vi "DrawSurface.vi"(0 "Surface":T1={"Row Interval"=1.0, "Col Interval"=1.0, "Base"=1.0, "Color Box"=1703680, "Alpha"=1.0}, 1 "Name":string="Surface", 2 "path":path, 3 "error in (no error)":errorcluster) -> (5 "object out":refnum<vi>, 7 "error out":errorcluster)   [LabVIEW 2017]
uses:
  <vilib>/picture/3D Picture Control/Object/Create Object (name).vi
  <vilib>/picture/3D Picture Control/NI_3D Picture Control.lvlib
panel:
  out "Color":T2={"Red"=1.0, "Green"=0.0, "Blue"=0.0, "Alpha"=1.0}
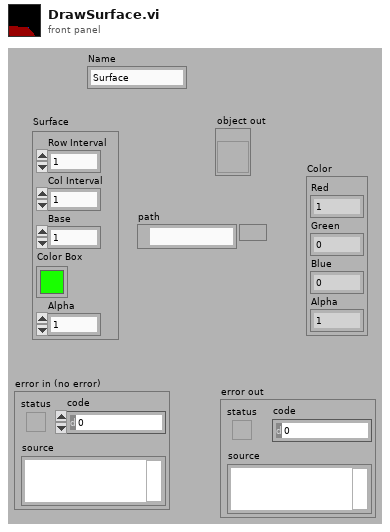
[diagram p1: front panel]
types:
  T1 = cluster{"Row Interval":sgl, "Col Interval":sgl, "Base":sgl, "Color Box":u32, "Alpha":sgl}
  T2 = cluster{"Red":sgl, "Green":sgl, "Blue":sgl, "Alpha":sgl}
  T3 = typedef "QT_Image.ctl" = cluster{"Width":i32, "Height":i32, "Depth":i32, "data":u8[], "Compressed data":u8[], "Color table":u32[], "Duration":i32, "Options":i32, "Timestamp":i32, "ID":i32, "Reserved":i32, "Dialogs":u32}
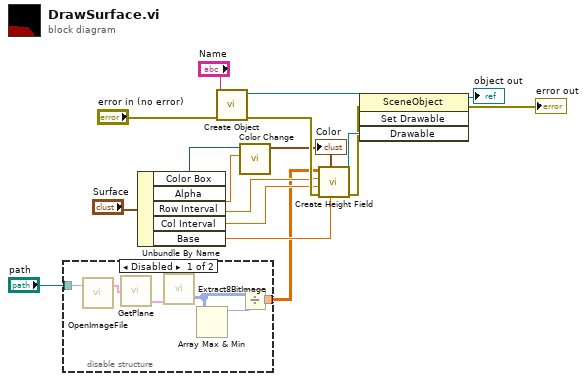
[diagram p0: block diagram]
diagram:
  n1 = disable-structure shown="Disabled" {
    disable-tunnel: [w19 _] -> w2
    disable-tunnel: "path" -> [w18 _]
    frame Disabled {
      n2 = call <userlib>:"OpenImageFile.vi"("selected path"=w18) -> ("Image Out"=w23:T3)  [unwired: 2 in]
      n3 = call <userlib>:"GetPlane.vi"("Image In"=w23) -> ("Blue Plane Out"=w20:T3)  [unwired: 2 out]
      n4 = call <userlib>:"Extract8BitImage.vi"("Image in"=w20) -> ("Intensity Graph"=w22:u8[][])  [unwired: 1 in, 1 out]
      n5 = Array Max & Min(array=w22) -> (max value=w21:u8)  [unwired: 3 out]
      n6 = Divide(x=w22, y=w21) -> (x/y=w19:dbl[][])
    }
    frame Enabled {
    }
  }
  n7 = Unbundle By Name("Surface") -> ("Color Box"=w10:u32, "Alpha"=w9:sgl, "Row Interval"=w5:sgl, "Col Interval"=w4:sgl, "Base"=w3:sgl)
  n8 = call-poly <vilib>:"Create Object.vi"("error in (no error)"="error in (no error)", "Name"="Name") -> ("error out"=w12:errorcluster, "Scene:New Object"=w15:refnum<vi>)  [unwired: 8 in]
  n9 = call <vilib>:"Color Change.vi"("Alpha"=w9, "Color"=w10) -> ("RGBA"=w8:cluster{"R":sgl, "G":sgl, "B":sgl, "A":sgl})  [unwired: 9 in]
  "Color" <- w8
  n10 = call <vilib>:"Create Height Field.vi"("Base Height"=w3, "Color"=w8, "error in (no error)"=w12, "Column Interval"=w4, "Row Interval"=w5, "Data"=w2) -> ("error out"=w11:errorcluster, "New Height Field Refnum"=w16:refnum<vi>)  [unwired: 4 in]
  n11 = invoke class="SceneObject" method="Set Drawable"(reference=w15, error in=w11, "Drawable"=w16) -> (reference out=→"object out":refnum<vi>, error out=→"error out":errorcluster)  [unwired: 1 in, 2 out]
